vi "rwfm_CreateChan.vi"(8 "error in":errorcluster, 9 "Total Avail Channels":i32, 10 "Sensitivity":sgl[](array[numeric]), 11 "Dynamic FPGA VI Reference":T1) -> (0 "error out":errorcluster, 3 "Dynamic FPGA VI Reference":T1)   [LabVIEW 2015]
doc: "This VI collects and sends scaling coefficients as well as channel count to the FPGA. The number of elements in \"Channel Info\" must equal the number of channels acquired by the FPGA."
uses:
  <vilib>/addons/InsightCM/Devices/Shared/cRIOWfmAcq/subVIs/RIO Wfm Cust Ctrls/rwfm_DynamicFPGAref2.ctl
  <vilib>/Utility/error.llb/Error Cluster From Error Code.vi
  <vilib>/rvi/errors/niLvFpgaAdjustHostInterfaceError.vi
  <vilib>/rvi/interface/nirviReadWriteControl/nirviReadWriteControl.xnode
  <vilib>/addons/InsightCM/Devices/Shared/cRIOWfmAcq/cRIOWfmLib.lvlib
  <vilib>/rvi/interface/Simulation/niFpgaSimulationCallBeginRW.vi
  NiFpgaLv.dll
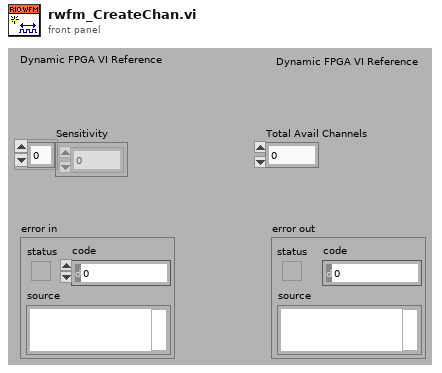
[diagram p1: front panel]
types:
  T1 = typedef "cRIOWfmLib.lvlib/rwfm_DynamicFPGAref2.ctl" = refnum<k20>
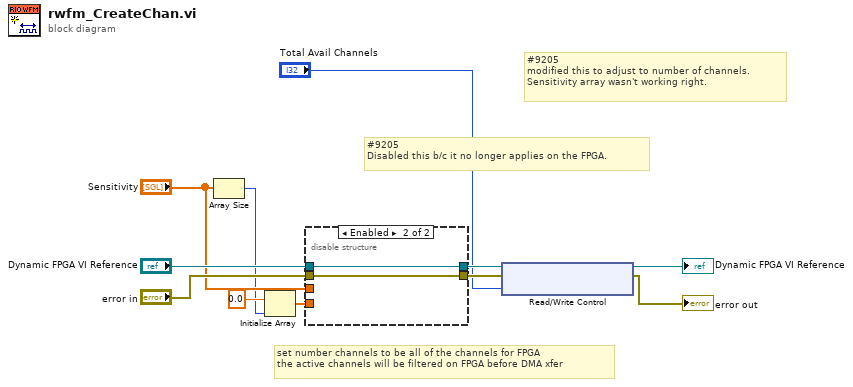
[diagram p0: block diagram]
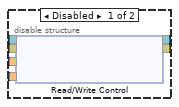
[diagram p2: hidden frame]
diagram:
  # "#9205\nmodified this to adjust to number of channels.\nSensitivity array wasn't working right."
  # "#9205\nDisabled this b/c it no longer applies on the FPGA."
  # "set number channels to be all of the channels for FPGA\nthe active channels will be filtered on FPGA before DMA xfer"
  n1 = Array Size(array="Sensitivity") -> (size(s)=w2:i32)
  n2 = Initialize Array(sgl 0.0, w2) -> (w5:sgl[])
  n3 = disable-structure shown="Enabled" {
    disable-tunnel: [w17 w18] -> w10
    disable-tunnel: [w16 w19] -> w9
    disable-tunnel: "error in" -> [w15 w19]
    disable-tunnel: "Dynamic FPGA VI Reference" -> [w14 w18]
    disable-tunnel: w5 -> [w13 _]
    disable-tunnel: "Sensitivity" -> [w12 _]
    frame Disabled {
      n4 = xnode "Read/Write Control"("FPGA VI Reference In"=w14, "error in"=w15, "Custom Scale Slope"=w12, "Custom Scale Intercept"=w13) -> ("FPGA VI Reference Out"=w17:T1, "error out"=w16:errorcluster)
    }
    frame Enabled {
    }
  }
  n5 = xnode "Read/Write Control"("FPGA VI Reference In"=w10, "error in"=w9, "Total Avail Channels"="Total Avail Channels") -> ("FPGA VI Reference Out"=→"Dynamic FPGA VI Reference":T1, "error out"=→"error out":errorcluster)
